vi "MaeanderDemo_Dlg.vi"(8 "error in (no error)":errorcluster) -> (0 "error out":errorcluster, 2 "Maeander Parameter":T1={"Number"=5, "X Start"=0.0, "Y Start"=0.0, "X Size"=2.0, "Y Size"=20.0} {"Y Size" format="%.6f"; "X Size" format="%.6f"; "Y Start" format="%.6f"; "X Start" format="%.6f"}, 3 "OK Out":bool)   [LabVIEW 2018, in "TangoOWN.lvlib"]
uses:
  TangoOWN.lvlib
  Maeander_Param.ctl
panel:
  in  "Cancel":bool caption="Stop"
  in  "OK":bool
  in  "X Size":dbl=2.0 format="%.6f"
  in  "Y Size":dbl=20.0 format="%.6f"
  in  "Y Start":dbl format="%.6f"
  in  "X Start":dbl format="%.6f"
  in  "Number":i32=5
  out "XY Graph":cluster{dbl, dbl}[](graph)
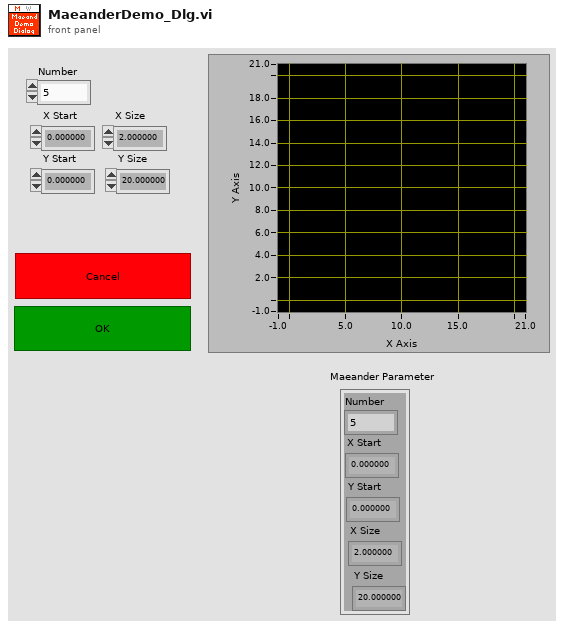
[diagram p1: front panel]
types:
  T1 = typedef "TangoOWN.lvlib/Maeander_Param.ctl" = cluster{"Number":i32, "X Start":dbl, "Y Start":dbl, "X Size":dbl, "Y Size":dbl}
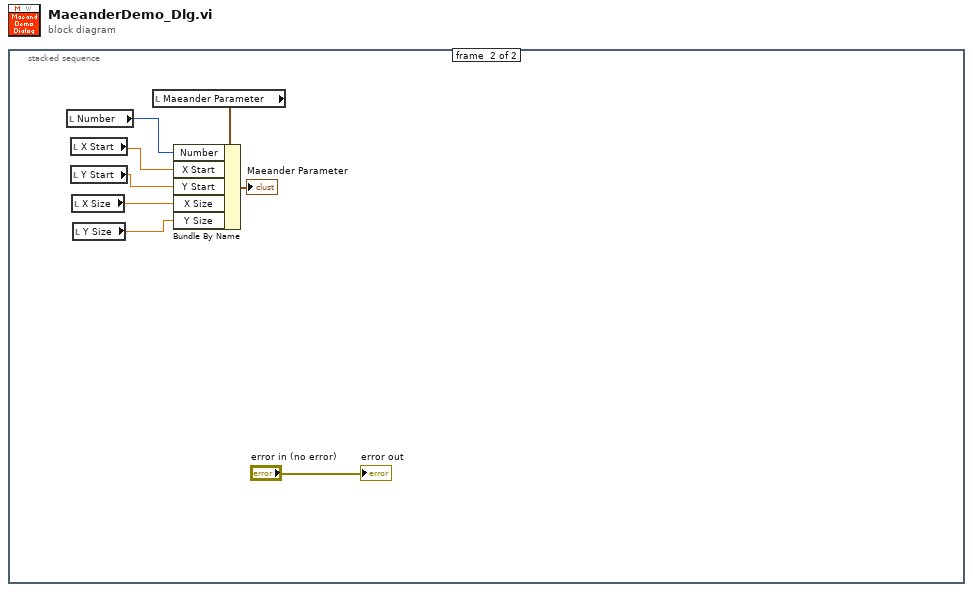
[diagram p0: block diagram]
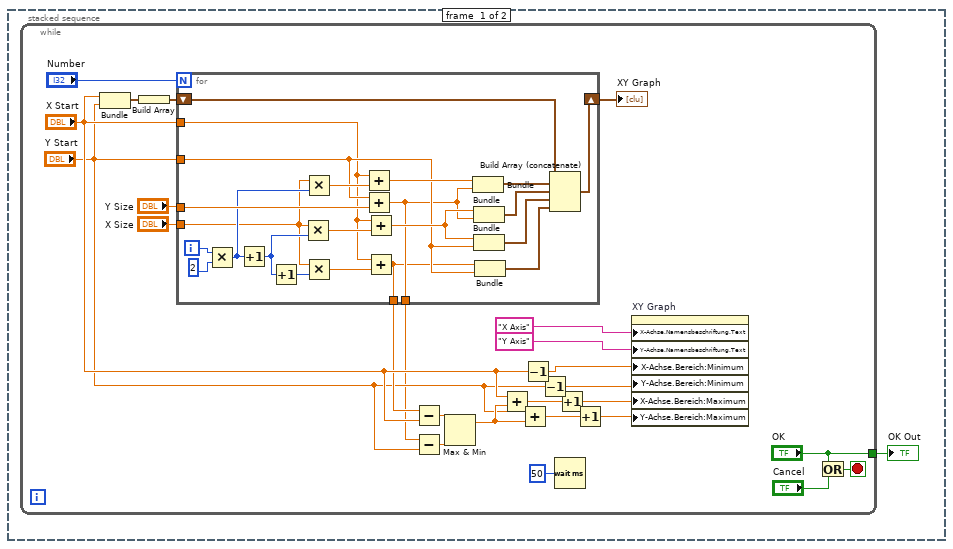
[diagram p2: hidden frame]
diagram:
  n1 = stacked-sequence {
    frame #0 {
      n2 = while {
        tunnel: ["OK"] -> w1
        stop <- w13 stop-if-true
        n3 = Bundle("X Start"="X Start", "Y Start"="Y Start") -> (w20:cluster{"X Start":dbl, "Y Start":dbl})  [unwired: 1 in]
        n4 = Build Array(w20) -> (w19:cluster{"X Start":dbl, "Y Start":dbl}[])
        n5 = for {
          N: "Number" -> [_]
          tunnel: "Y Size" -> [w48]
          tunnel: "Y Start" -> [w35]
          tunnel: "X Start" -> [w29]
          tunnel: "X Size" -> [w32]
          shift-right: [w46] -> w21
          shift-left: w19 -> [w45]
          tunnel: [w30] -> w4
          tunnel: [w27] -> w7
          i -> [w42]
          n6 = Multiply(x=w42, y=2) -> (x*y=w40:i32)
          n7 = Increment(x=w40) -> (x+1=w34:i32)
          n8 = Increment(x=w34) -> (x+1=w31:i32)
          n9 = Multiply(x=w32, y=w34) -> (x*y=w33:dbl)
          n10 = Multiply(x=w32, y=w40) -> (x*y=w41:dbl)
          n11 = Multiply(x=w32, y=w31) -> (x*y=w28:dbl)
          n12 = Add(x=w29, y=w41) -> (x+y=w38:dbl)
          n13 = Add(x=w35, y=w48) -> (x+y=w30:dbl)
          n14 = Add(x=w29, y=w33) -> (x+y=w47:dbl)
          n15 = Add(x=w29, y=w28) -> (x+y=w27:dbl)
          n16 = Bundle(w38, w30) -> (w37:cluster{dbl, dbl})  [unwired: 1 in]
          n17 = Bundle(w47, w30) -> (w44:cluster{dbl, dbl})  [unwired: 1 in]
          n18 = Bundle(w47, "Y Start"=w35) -> (w43:cluster{dbl, "Y Start":dbl})  [unwired: 1 in]
          n19 = Bundle(w27, "Y Start"=w35) -> (w36:cluster{dbl, "Y Start":dbl})  [unwired: 1 in]
          n20 = Build Array (concatenate)(w45, w37, w44, w43, w36) -> (w46:cluster{"X Start":dbl, "Y Start":dbl}[])
        }
        "XY Graph" <- w21
        n21 = Subtract(x=w7, y="X Start") -> (x-y=w11:dbl)
        n22 = Subtract(x=w4, y="Y Start") -> (x-y=w10:dbl)
        n23 = Max & Min(x=w11, y=w10) -> (max(x,y)=w8:dbl)  [unwired: 1 out]
        n24 = Add(x="X Start", y=w8) -> (x+y=w6:dbl)
        n25 = Add(x="Y Start", y=w8) -> (x+y=w3:dbl)
        n26 = Decrement(x="X Start") -> (x-1=w18:dbl)
        n27 = Decrement(x="Y Start") -> (x-1=w17:dbl)
        n28 = Wait (ms)(milliseconds to wait=u32 50) -> ()  [unwired: 1 out]
        n29 = Increment(x=w6) -> (x+1=w16:dbl)
        n30 = Increment(x=w3) -> (x+1=w15:dbl)
        n31 = property on="XY Graph" class="XYGraph (strict)"("X-Achse.Namensbeschriftung.Text"="X Axis" ("X Scale.Name Label.Text"), "Y-Achse.Namensbeschriftung.Text"="Y Axis" ("Y Scale.Name Label.Text"), "X-Achse.Bereich:Minimum"=w18, "Y-Achse.Bereich:Minimum"=w17, "X-Achse.Bereich:Maximum"=w16, "Y-Achse.Bereich:Maximum"=w15) -> ()  [unwired: 2 in, 2 out]
        n32 = Or(x="OK", y="Cancel") -> (x .or. y?=w13:bool)
      }
      "OK Out" <- w1
    }
    frame #1 {
      n33 = local read "Number"() -> (w52:i32)
      n34 = local read "X Start"() -> (w51:dbl)
      n35 = local read "Y Start"() -> (w50:dbl)
      n36 = local read "X Size"() -> (w49:dbl)
      n37 = local read "Y Size"() -> (w53:dbl)
      n38 = local read "Maeander Parameter"() -> (w54:T1)
      n39 = Bundle By Name(cluster=w54, "Number"=w52, "X Start"=w51, "Y Start"=w50, "X Size"=w49, "Y Size"=w53) -> (→"Maeander Parameter":T1)
      "error out" <- "error in (no error)"
    }
  }
